vi "CheckPasserState.vi"(8 "error in (no error)":errorcluster, 10 "GameRef":refnum<data-value>, 11 "object in":refnum<class "SupportAttackerRole.lvclass">) -> (0 "error out":errorcluster, 2 "searchTarget":bool=TRUE, 3 "object out":refnum<class "SupportAttackerRole.lvclass">)   [LabVIEW 2023, in "SupportAttackerRole.lvclass"]
uses:
  SupportAttackerRole.lvclass
  Game_class/Game.lvclass
  Robot_class/roles.ctl
  Game_class/Game.lvclass/Game.ctl
  Team_class/Team.lvclass/Team.ctl
  PrimaryAttacker_class/PrimaryAttackerRole_states.ctl
  Game_class/Read OffensiveTeam.vi
  Team_class/Read RobotRef.vi
  Ally_class/Ally.lvclass
  C:/Users/ebert/Documents/codes/SSL/repo/SSL_AI/Team_class/Team.lvclass
  Robot_class/Robot.lvclass
  NewSTP/NewRoles/Role_v2_class/Role_v2.lvclass
  Utilities_class/Utilities.lvclass
  PrimaryAttacker_class/PrimaryAttackerRole.lvclass
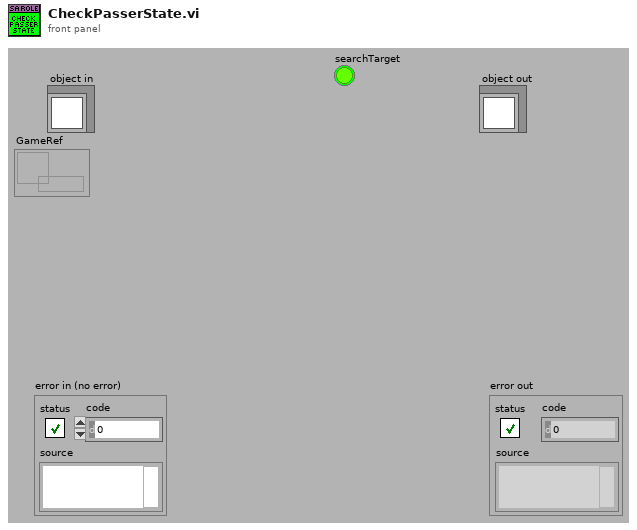
[diagram p1: front panel]
types:
  T1 = typedef "roles.ctl" = enum16{"SimpleBallPlacement", "BallPlacementAllyPasser", "BallPlacementAllyReceiver", "BallPlacementEnemy", "5Robots5th", "PassBestReceiver", "5Robots4th", "5Robots3rd", "5Robots2nd", "5Robots1st", "PassBestRobot", "WaitPass", "ABCThirdKicker", "ABCFirstKicker", "ABCSecondKicker", "Tabler", "TableFinalizer", "PrepareRollToPassRoller", "PrepareRollToPassReceiver", "SimplePassRoll", "SimplePassRollReceiver", "PenaltyDefense", "PreparePassReceiver 2", "PreparePassReceiver 1", "PassObserver", "Timeout", "Goto", "ZigZag", "None", "BallOutOfField", "DefenderArea", "Duelist", "AttackerStop", "FollowAttacker", "KeeperRole", "KickPenalty", "AttackerAimGoal", "AttackerBlock", "Marker", "Halt", "Shoot", "PassKicker", "PassReceiver", "TestRole", "PenaltyAttacker", "PrimaryAttackerRole", "SupportAttackerRole"}
  T2 = typedef "PrimaryAttackerRole.lvclass/PrimaryAttackerRole_states.ctl" = enum16{"Intercept", "PrepareShot", "Shoot", "Pass"}
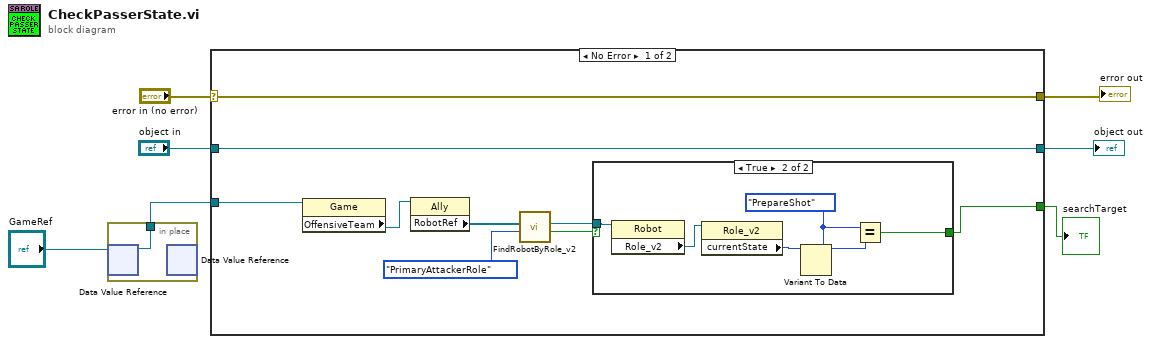
[diagram p0: block diagram]
diagram:
  n1 = in-place {
    in-place-border: [w8] -> w2
    n2 = in-place-dvr #1("GameRef") -> (w8:refnum<class "Game.lvclass">)  [unwired: 1 out]
    n3 = in-place-dvr #1() -> ()  [unwired: 1 in, 2 out]
  }
  n4 = case shown="No Error" "error in (no error)" {
    selector: "error in (no error)" -> [w17 w26]
    tunnel: [w17 w26] -> w6
    tunnel: [w16 w25] -> w4
    tunnel: "object in" -> [w16 w25]
    tunnel: w2 -> [w11 _]
    tunnel: [w9 _] -> w1
    frame No Error {
      n5 = property class="Game"(reference=w11) -> ("OffensiveTeam"=w15:refnum<class "Ally.lvclass">)  [unwired: 1 in, 2 out]
      n6 = property class="Ally"(reference=w15) -> ("RobotRef"=w14:refnum<class "Robot.lvclass">[])  [unwired: 1 in, 2 out]
      n7 = call "FindRobotByRole_v2.vi"("role"=roles."PrimaryAttackerRole", "Array"=w14) -> ("foundRobot"=w10:bool, "Robot"=w12:refnum<class "Robot.lvclass">)  [unwired: 6 in, 2 out]
      n8 = case shown="True" w10 {
        selector: w10 -> [w18 _]
        tunnel: w12 -> [_ w24]
        tunnel: [w18 w22] -> w9
        frame False {
        }
        frame True {
          w20 = PrimaryAttackerRole_states."PrepareShot" ("Enum")
          n9 = property class="Robot"(reference=w24) -> ("Role_v2"=w23:refnum<class "Role_v2.lvclass">)  [unwired: 1 in, 2 out]
          n10 = property class="Role_v2"(reference=w23) -> ("currentState"=w21:u8)  [unwired: 1 in, 2 out]
          n11 = Variant To Data(type=w20, Variant=w21) -> (data=w19:T2)  [unwired: 1 in, 1 out]
          n12 = Equal?(x=w20, y=w19) -> (x = y?=w22:bool)
        }
      }
    }
    frame Error {
    }
  }
  "error out" <- w6
  "object out" <- w4
  "searchTarget" <- w1
